vi "Check Byte Align.vi"() -> ()   [LabVIEW 2012]
uses:
  demo dll.dll
panel:
  out "size of cluster":u32
  in  "TestAlign":T1
  out "size of struct":i32
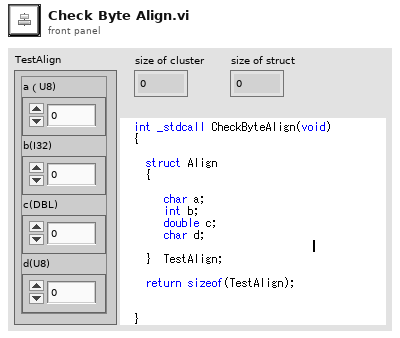
[diagram p1: front panel]
types:
  T1 = cluster{"a（U8)":u8, "b(I32)":i32, "c(DBL)":dbl, "d(U8)":u8}
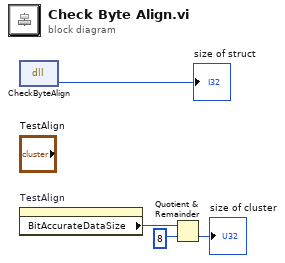
[diagram p0: block diagram]
diagram:
  n1 = dll-call lib="PTH1+abs EBOOK\t功能块DLLdemo dll.dll" fn="CheckByteAlign"() -> ("返回类型"=→"size of struct":i32)  [unwired: 3 in, 2 out]
  n2 = property on="TestAlign" class="Clust (严格)"() -> ("BitAccurateDataSize"=w3:u32)  [unwired: 2 in, 2 out]
  n3 = Quotient & Remainder(x=w3, y=u32 8) -> (floor(x/y)=→"size of cluster":u32)  [unwired: 1 out]
